vi "Clear Task.vi"(8 "error in":errorcluster, 11 "NI PWM Output in":refnum<class "NI PWM Output.lvclass">) -> (0 "error out":errorcluster, 3 "NI PWM Output out":refnum<class "NI PWM Output.lvclass">)   [LabVIEW 2023, in "HardwareAbstractionLayer_LVOOP.lvlib" / "NI PWM Output.lvclass"]
doc: "DAQ AO Clear Data"
uses:
  NI PWM Output.lvclass
  NI PWM Output.lvclass/NI PWM Output.ctl
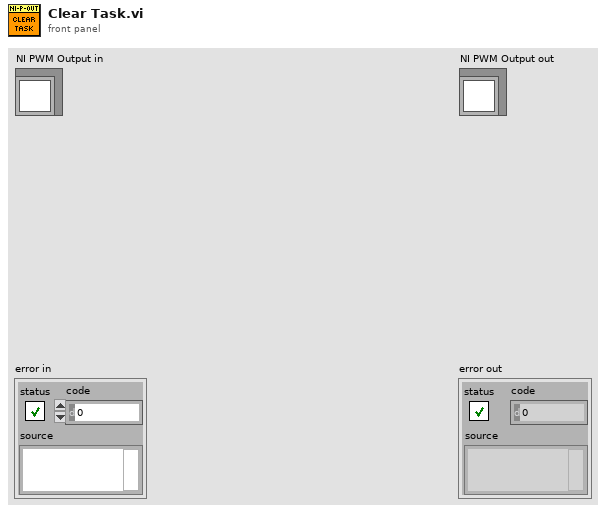
[diagram p1: front panel]
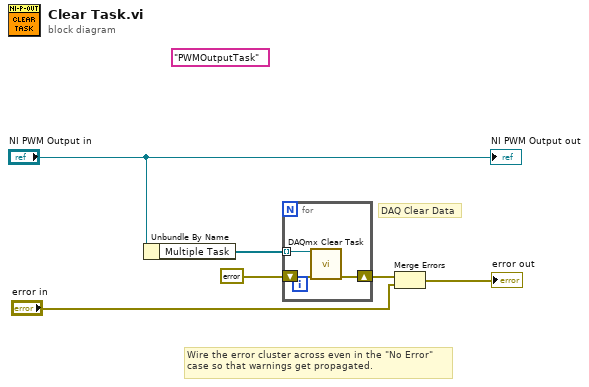
[diagram p0: block diagram]
diagram:
  (unwired) "PWMOutputTask" ("new task name")
  # "DAQ Clear Data"
  # "Wire the error cluster across even in the \"No Error\"\ncase so that warnings get propagated."
  n1 = Unbundle By Name("NI PWM Output in") -> ("Multiple Task"=w1:refnum<k21>[])
  n2 = for {
    shift-right: [w9] -> w6
    shift-left: errorcluster {"status"=FALSE, "code"=0, "source"=""} ("error in") -> [w8]
    tunnel: w1 -> [w7] mode=indexing
    n3 = call <vilib>:"DAQmx Clear Task.vi"("task in"=w7, "error in"=w8) -> ("error out"=w9:errorcluster)  [unwired: 13 in]
  }
  n4 = Merge Errors(w6, "error in") -> (→"error out":errorcluster)
  "NI PWM Output out" <- "NI PWM Output in"
